vi "GetTemperature.vi"(8 "error in (no error)":errorcluster, 9 "Instrument Ref In":refnum<k24>) -> (0 "Temperature\nStatus":i32(ring) items=["TemperatureUnknown"=0, "Stable"=1, "Tracking"=2, "Near"=5, "Chasing"=6, "Filling"=7, "Standby"=10, "Disabled"=13, "ImpedanceNotFunction"=14, "TempFailure"=15], 1 "Temperature":dbl, 2 "error out":errorcluster, 3 "Instrument Ref Out":refnum<k24>, 4 "GetTemperature Error":i32)   [LabVIEW 2016]
uses:
  C:/user/repos/levylab_inst_ppms2/lvsrc/QDInstrument_LabView/QDInstrument.dll
  QDInstrument.dll
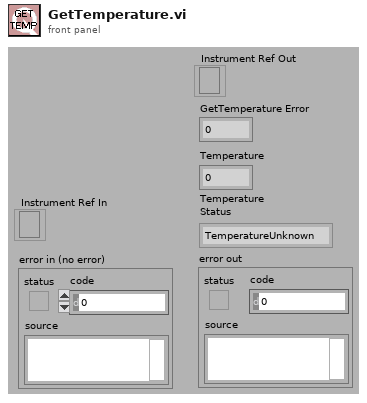
[diagram p1: front panel]
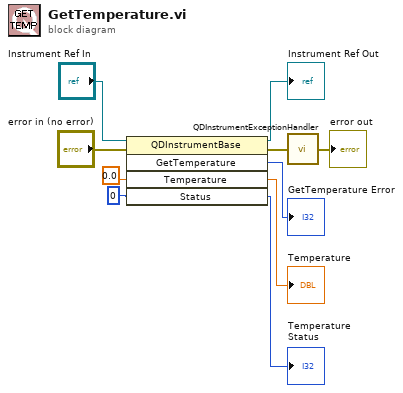
[diagram p0: block diagram]
diagram:
  n1 = invoke class="QDInstrumentBase" method="GetTemperature"(reference="Instrument Ref In", error in="error in (no error)", "Temperature"=0.0, "Status"=0) -> (reference out=→"Instrument Ref Out":refnum<k24>, error out=w2:errorcluster, "GetTemperature"=→"GetTemperature Error":i32, "Temperature"=→"Temperature":dbl, "Status"=→"Temperature\nStatus":i32)  [unwired: 1 in]
  n2 = call "QDInstrumentExceptionHandler.vi"("Error in"=w2) -> ("Error out"=→"error out":errorcluster)
